vi "Set Button Attribute.vi"(8 "error in (no error)":errorcluster, 10 "Button Attribute":T1, 11 "QMenu Class in":refnum<class "QMenu Class.lvclass">) -> (0 "error out":errorcluster, 3 "QMenu Class out":refnum<class "QMenu Class.lvclass">)   [LabVIEW 2020, in "QTab.lvlib" / "QMenu Class.lvclass"]
uses:
  QMenu Class.lvclass
  Button Attribute.ctl
  Command.ctl
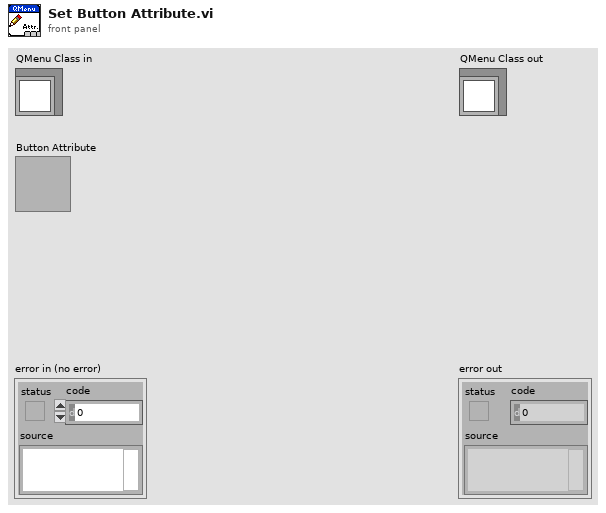
[diagram p1: front panel]
types:
  T1 = typedef "QTab.lvlib/QMenu Class.lvclass/Button Attribute.ctl" = cluster{"Label":string, "Button Text":string, "Closable":bool, "Draggable":bool}
  T2 = typedef "QTab.lvlib/QMenu Class.lvclass/Command.ctl" = enum16{"Initialize", "Get Active Button", "Set Active Button", "Set Button Attribute", "Add Button", "Close Button", "Draw", "Stop"}
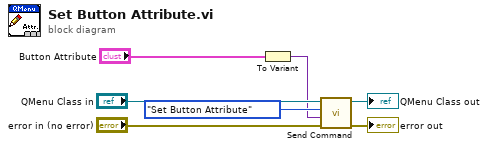
[diagram p0: block diagram]
diagram:
  n1 = To Variant(anything="Button Attribute") -> (Variant=w3:variant)
  n2 = call "Send Command.vi"("error in (no error)"="error in (no error)", "Data"=w3, "Command"=Command."Set Button Attribute", "QMenu Class in"="QMenu Class in") -> ("error out"=→"error out":errorcluster, "QMenu Class out"=→"QMenu Class out":refnum<class "QMenu Class.lvclass">)  [unwired: 6 in]
